vi "PiVision.vi"(11 "Port":u16=8622) -> ()   [LabVIEW 2014]
uses:
  Vision Data.vi
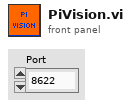
[diagram p1: front panel]
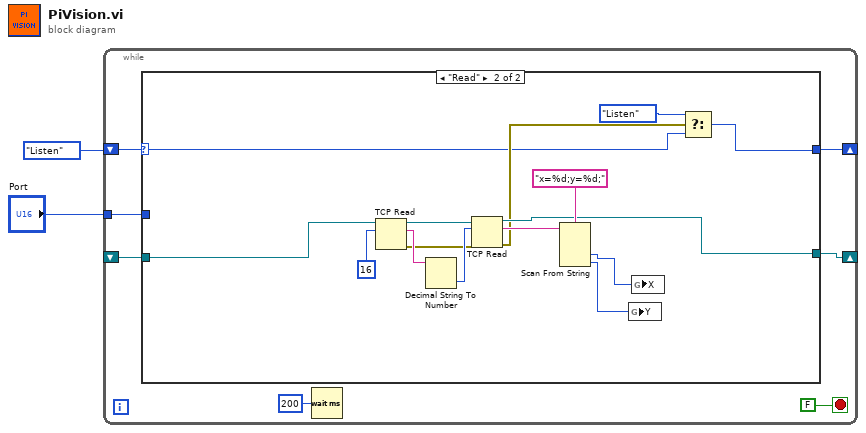
[diagram p0: block diagram]
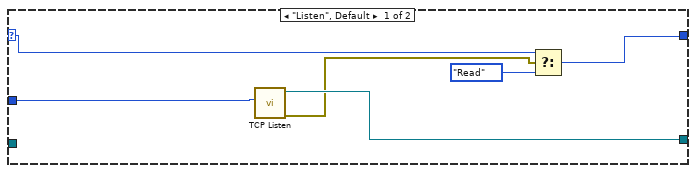
[diagram p2: hidden frame]
diagram:
  n1 = while {
    shift-right: [w7] -> _
    shift-left: enum16{"Listen", "Read"}."Listen" -> [w8]
    tunnel: "Port" -> [w6]
    shift-right: [w5] -> _
    shift-left: _ -> [w4]
    stop <- FALSE stop-if-true
    n2 = case shown="\"Read\"" w8 {
      selector: w8 -> [w11 w19]
      tunnel: [w13 w18] -> w7
      tunnel: w6 -> [w15 _]
      tunnel: [w14 w22] -> w5
      tunnel: w4 -> [_ w23]
      frame "Listen", Default {
        n3 = call <vilib>:"TCP Listen.vi"("port"=w15) -> ("error out"=w12:errorcluster, "connection ID"=w14:refnum<k5>)  [unwired: 6 in, 3 out]
        n4 = Select(t=w11, s=w12, f=enum16{"Listen", "Read"}."Read") -> (s? t:f=w13:enum16{"Listen", "Read"})
      }
      frame "Read" {
        n5 = TCP Read(connection ID=w23, bytes to read=16) -> (connection ID out=w27:refnum<k5>, data out=w29:string, error out=w26:errorcluster)  [unwired: 3 in]
        n6 = Decimal String To Number(string=w29) -> (number=w28:i32)  [unwired: 2 in, 1 out]
        n7 = TCP Read(connection ID=w27, bytes to read=w28, error in (no error)=w26) -> (connection ID out=w22:refnum<k5>, data out=w24:string, error out=w20:errorcluster)  [unwired: 2 in]
        n8 = Scan From String(format string="x=%d;y=%d;", input string=w24) -> (output 1=w17:i32, output 2=w16:i32)  [unwired: 4 in, 3 out]
        n9 = global write "Vision Data.vi" "Y"(w16) -> ()
        n10 = global write "Vision Data.vi" "X"(w17) -> ()
        n11 = Select(t=enum16{"Listen", "Read"}."Listen", s=w20, f=w19) -> (s? t:f=w18:enum16{"Listen", "Read"})
      }
    }
    n12 = Wait (ms)(milliseconds to wait=u32 200) -> ()  [unwired: 1 out]
  }
